vi "Run.vi"(8 "error in (no error)":errorcluster, 10 "Maze (0: Empty, -1: Enemy. >0: Teammate":i32[][](array[numeric]), 11 "Wanderer in":refnum<class "Wanderer.lvclass">) -> (0 "error out":errorcluster, 1 "Direction":T1, 2 "Action":T2, 3 "Wanderer out":refnum<class "Wanderer.lvclass">)   [LabVIEW 2014, in "Wanderer.lvclass"]
uses:
  Wanderer.lvclass
  Action Enum.ctl
  Direction Enum.ctl
  Wanderer.lvclass/Wanderer.ctl
  Maze 2.0.lvclass
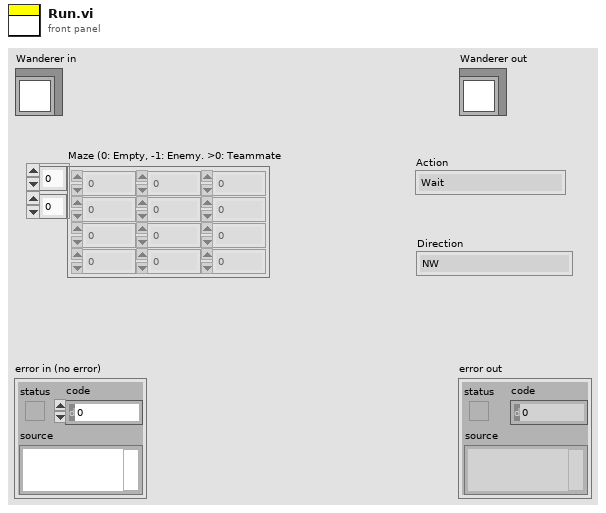
[diagram p1: front panel]
types:
  T1 = typedef "Maze 2.0.lvclass/Direction Enum.ctl" = enum16{"NW", "N", "NE", "E", "SE", "S", "SW", "W"}
  T2 = typedef "Maze 2.0.lvclass/Action Enum.ctl" = enum16{"Wait", "Move", "Attack", "Replicate"}
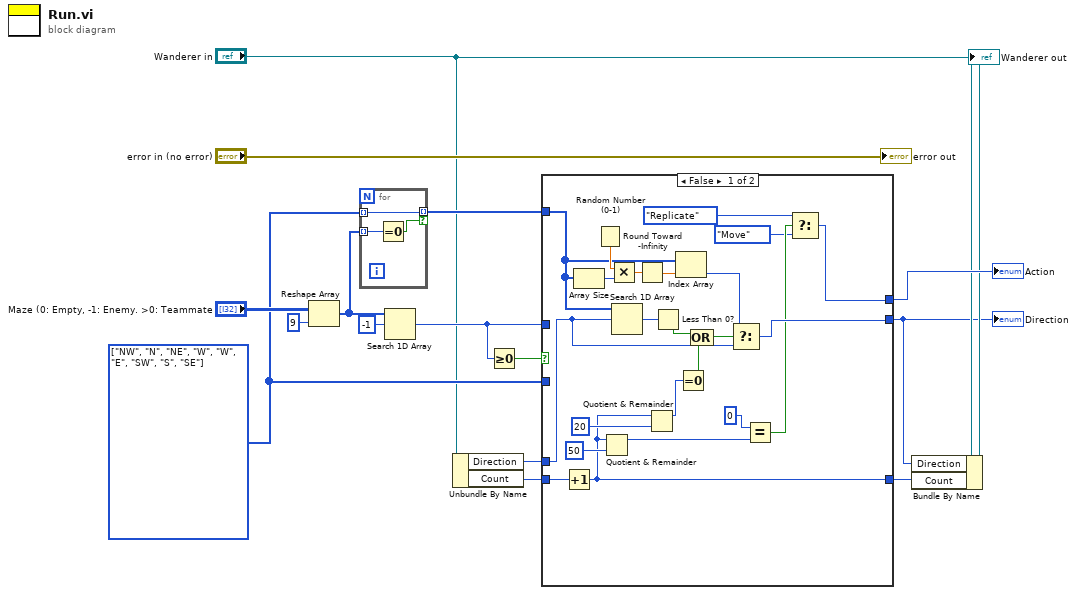
[diagram p0: block diagram]
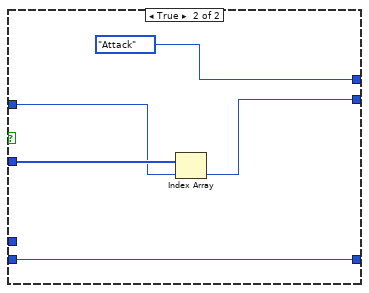
[diagram p2: hidden frame]
diagram:
  w9 = T1[] [enum."NW", enum."N", enum."NE", enum."W", enum."W", enum."E", enum."SW", enum."S", enum."SE"] items=["NW", "N", "NE", "E", "SE", "S", "SW", "W"]
  n1 = Reshape Array("Maze (0: Empty, -1: Enemy. >0: Teammate", 9 ("dimension size")) -> (w13:i32[])
  n2 = for {
    tunnel: w13 -> [w19] mode=indexing
    tunnel: w9 -> [w18] mode=indexing
    tunnel: [w18] -> w11 mode=indexing if=w17
    n3 = Equal To 0?(x=w19) -> (x = 0?=w17:bool)
  }
  n4 = Search 1D Array(1D array=w13, element=-1) -> (index of element=w12:i32)  [unwired: 1 in]
  n5 = Unbundle By Name("Wanderer in") -> ("Direction"=w2:T1, "Count"=w4:i32)
  n6 = Greater Or Equal To 0?(x=w12) -> (x >= 0?=w14:bool)
  n7 = case shown="False" w14 {
    tunnel: [w40 Action_Enum."Attack" ("Action")] -> w8
    tunnel: w12 -> [_ w46]
    tunnel: w9 -> [_ w47]
    tunnel: [w30 w45] -> w1
    tunnel: w11 -> [w28 _]
    tunnel: w4 -> [w22 w43]
    tunnel: [w21 w43] -> w3
    tunnel: w2 -> [w20 _]
    frame False {
      n8 = Increment(x=w22) -> (x+1=w21:i32)
      n9 = Array Size(array=w28) -> (size(s)=w38:i32)
      n10 = Random Number (0-1)() -> (number: 0 to 1=w39:dbl)
      n11 = Quotient & Remainder(x=w21, y=50 ("dimension size")) -> (x-y*floor(x/y)=w35:i32)  [unwired: 1 out]
      n12 = Multiply(x=w39, y=w38) -> (x*y=w29:dbl)
      n13 = Search 1D Array(1D array=w28, element=w20) -> (index of element=w37:i32)  [unwired: 1 in]
      n14 = Round Toward -Infinity(1:w29) -> (0:w27:dbl)
      n15 = Quotient & Remainder(x=w21, y=20 ("dimension size")) -> (x-y*floor(x/y)=w33:i32)  [unwired: 1 out]
      n16 = Less Than 0?(x=w37) -> (x < 0?=w36:bool)
      n17 = Index Array(array=w28, index=w27) -> (element=w26:T1)
      n18 = Equal To 0?(x=w33) -> (x = 0?=w32:bool)
      n19 = Compound Arithmetic op=OR(w36, w32) -> (w31:bool)
      n20 = Select(t=w26, s=w31, f=w20) -> (s? t:f=w30:T1)
      n21 = Equal?(x=0, y=w35) -> (x = y?=w25:bool)
      n22 = Select(t=Action_Enum."Replicate" ("Action"), s=w25, f=Action_Enum."Move" ("Action")) -> (s? t:f=w40:T2)
    }
    frame True {
      n23 = Index Array(array=w47, index=w46) -> (element=w45:T1)
    }
  }
  "Action" <- w8
  "Direction" <- w1
  n24 = Bundle By Name(cluster="Wanderer in", "Direction"=w1, "Count"=w3) -> (→"Wanderer out":refnum<class "Wanderer.lvclass">)
  "error out" <- "error in (no error)"
